vi "getMaxValue.vi"(8 "error in (no error)":errorcluster, 11 "IProperty in":refnum<class "IProperty.lvclass">) -> (0 "error out":errorcluster, 2 "Maximum out":i64, 3 "IProperty out":refnum<class "IProperty.lvclass">)   [LabVIEW 2022 SP3, in "openDAQ.lvlib" / "IBaseObject.lvlib" / "IProperty.lvlib" / "IProperty.lvclass"]
uses:
  <instrlib>/openDAQ/Public/Classes/IProperty/IProperty.lvclass
  <instrlib>/openDAQ/Public/Classes/IProperty/IProperty.lvclass/IProperty.ctl
  <instrlib>/openDAQ/Public/Classes/daqCoreTypes/INumber/INumber.lvclass
  <instrlib>/openDAQ/Binaries/Windows/x86/copendaq32.dll
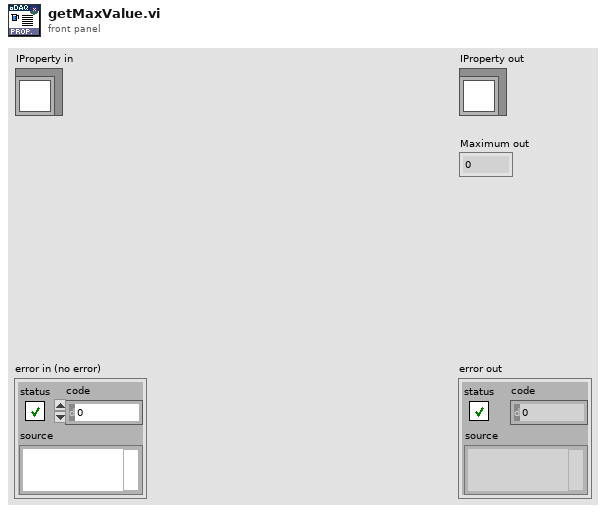
[diagram p1: front panel]
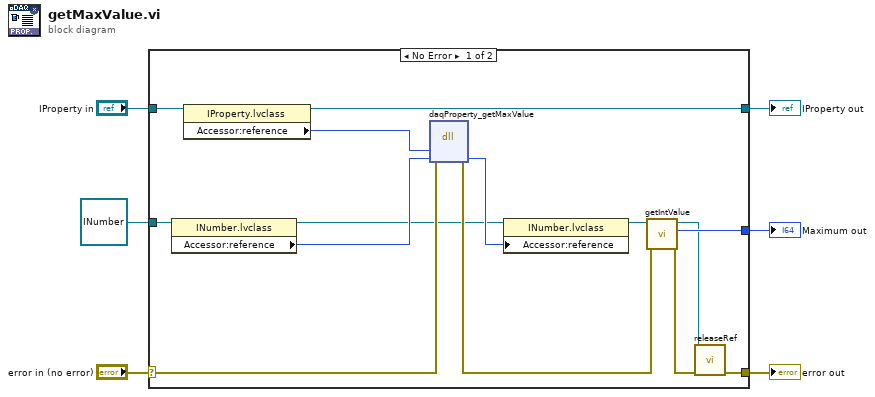
[diagram p0: block diagram]
diagram:
  n1 = case shown="No Error" "error in (no error)" {
    selector: "error in (no error)" -> [w16 w22]
    tunnel: [w9 w22] -> w5
    tunnel: [w15 w21] -> w3
    tunnel: "IProperty in" -> [w17 w21]
    tunnel: refnum<class "INumber.lvclass"> refnum ("openDAQ.lvlib:daqCoreTypes.lvlib:INumber.lvclass") -> [w13 _]
    tunnel: [w18 _] -> w1
    frame No Error {
      n2 = property class="INumber.lvclass"(reference=w13) -> (reference out=w11:refnum<class "INumber.lvclass">, "Accessor:reference"=w12:i64)  [unwired: 1 in, 1 out]
      n3 = property class="IProperty.lvclass"(reference=w17) -> (reference out=w15:refnum<class "IProperty.lvclass">, "Accessor:reference"=w14:i64)  [unwired: 1 in, 1 out]
      n4 = dll-call lib="C:/Program Files (x86)/National Instruments/LabVIEW 2022/instr.lib/openDAQ/Binaries/Windows/x86/copendaq*.*" fn="daqProperty_getMaxValue"(error in=w16, "property"=w14, "max"=w12) -> (error out=w19:errorcluster, "max"=w20:i64)  [unwired: 4 in, 1 out]
      n5 = property class="INumber.lvclass"(reference=w11, "Accessor:reference"=w20) -> (reference out=w10:refnum<class "INumber.lvclass">)  [unwired: 1 in, 1 out]
      n6 = call <instrlib>:"getIntValue.vi"("error in (no error)"=w19, "INumber in"=w10) -> ("error out"=w8:errorcluster, "Int Value out"=w18:i64, "INumber out"=w7:refnum<class "INumber.lvclass">)  [unwired: 7 in]
      n7 = call-dynamic "releaseRef.vi"("error in (no error)"=w8, "IBaseObject in"=w7) -> ("error out"=w9:errorcluster)  [unwired: 9 in]
    }
    frame Error {
    }
  }
  "error out" <- w5
  "IProperty out" <- w3
  "Maximum out" <- w1
